vi "DFD 2-Band Filter Bank Reconstruction with State.vi"   [LabVIEW 2017, in "NI_DigFilter_FilterBank.lvlib"]
doc: "Reconstructs signal from <B>lowpass channel</B> and <B>highpass channel</B> using a 2-band synthesis bank specified by <B>synthesis bank</B>. You must specify the most recent internal input states <B>state in</B> to get the correct output. \n\n<B>state out</B> contains the most recent internal output states, which can be used as <B>state in</B> for next call to this VI if you want to process the data continuously.\n\nThis VI is a polymorphic VI. The input data can be array or waveform data type.\n\nYou can call the VIs in <B>Filter Bank Design</B> sub-palette to design a filter bank."
uses:
  <vilib>/addons/Digital Filter Design/NI_DigFilter_FilterBank.lvlib
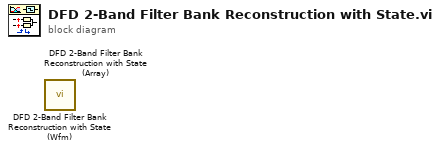
[diagram p0: block diagram]
diagram:
  n1 = call <vilib>:"DFD 2-Band Filter Bank Reconstruction with State (Wfm).vi"() -> ()  [unwired: 9 in, 3 out]
  n2 = call <vilib>:"DFD 2-Band Filter Bank Reconstruction with State (Array).vi"() -> ()  [unwired: 9 in, 3 out]
